vi "PointerToString.vi"(3 "stringpointer":i32 format="%.0x") -> (0 "string":string)   [LabVIEW 2011]
doc: "Gets the string at the memory pointer.\nCompare with StringToPointer.vi\n\nW.K. Walstra, © AIR Technical Automation bv\nwww.air.nl / info@air.nl (general info) / wiebe@air.nl (specific info)"
uses:
  KERNEL32.DLL
panel:
  # "nnnnn   nnn nnnnnn  \nnnnnnnn nnn nnnnnnn\nnnnnnnn nnn nnnnnnn\nnnnqnnn nnn nnn  nnn\nnnn  nnn nnn nnnnnnn\nnnn  nnn nnn nnnnnn  \nnnnnnnn nnn nnnnnnn\nnnnnnnn nnn nnn  nnn\nnnnnnnn nnn nnn  nnn\nnnn  nnn nnn nnn  nnn\nnnn  nnn nnn nnn  nnn"
  # "Technical Automation"
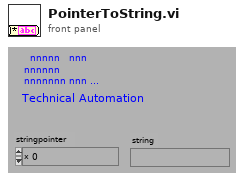
[diagram p1: front panel]
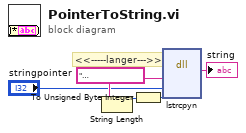
[diagram p0: block diagram]
diagram:
  w5 = "                                                                                                                                                                                                                                                              "
  # "<<-----langer--->>"
  n1 = String Length(string=w5) -> (length=w4:i32)
  n2 = To Unsigned Byte Integer(number=w4) -> (unsigned 8bit integer=w1:u8)
  n3 = dll-call lib="KERNEL32.DLL" fn="lstrcpyn"(w5, "stringpointer", w1) -> (→"string":string)  [unwired: 5 in, 3 out]
